vi "USS9804_ReadAD.vi"(8 "Error In":errorcluster, 10 "pBuf":u16[](array[numeric]), 11 "Handle":u64) -> (0 "Error Out":errorcluster, 2 "pBuf 2":u16[](array[numeric]), 3 "Handle 2":u64)   [LabVIEW 2015]
uses:
  USS9804.DLL
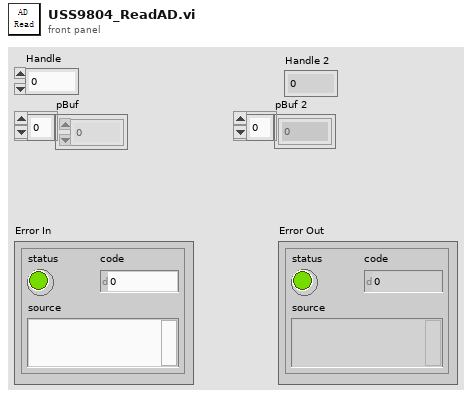
[diagram p1: front panel]
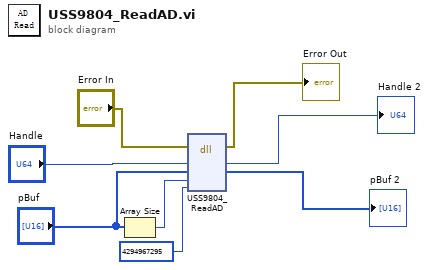
[diagram p0: block diagram]
diagram:
  n1 = Array Size(array="pBuf") -> (size(s)=w3:i32)
  n2 = dll-call lib="PTH2Sabs CYexinrongWorkplace\t普密斯Thickness-measurementLabVIEWUSS9804.DLL" fn="USS9804_ReadAD"(error in="Error In", "Handle"="Handle", "pBuf"="pBuf", "nCount"=w3, "timeout"=u32 4294967295) -> (error out=→"Error Out":errorcluster, "Handle"=→"Handle 2":u64, "pBuf"=→"pBuf 2":u16[])  [unwired: 5 in, 1 out]
